vi "CC Quad Image Viewer.vi"(11 "Files":path[](array[path])) -> ()   [LabVIEW 2024]
uses:
  <vilib>/Utility/miscctls.llb/LVCursorListTypeDef.ctl
panel:
  in  "Transpose 1":bool
  out "Detector 1":sgl[][](graph)
  in  "Transpose 3":bool
  out "Detector 3":sgl[][](graph)
  in  "Transpose 2":bool
  out "Detector 2":sgl[][](graph)
  in  "Transpose 4":bool
  out "Detector 4":sgl[][](graph)
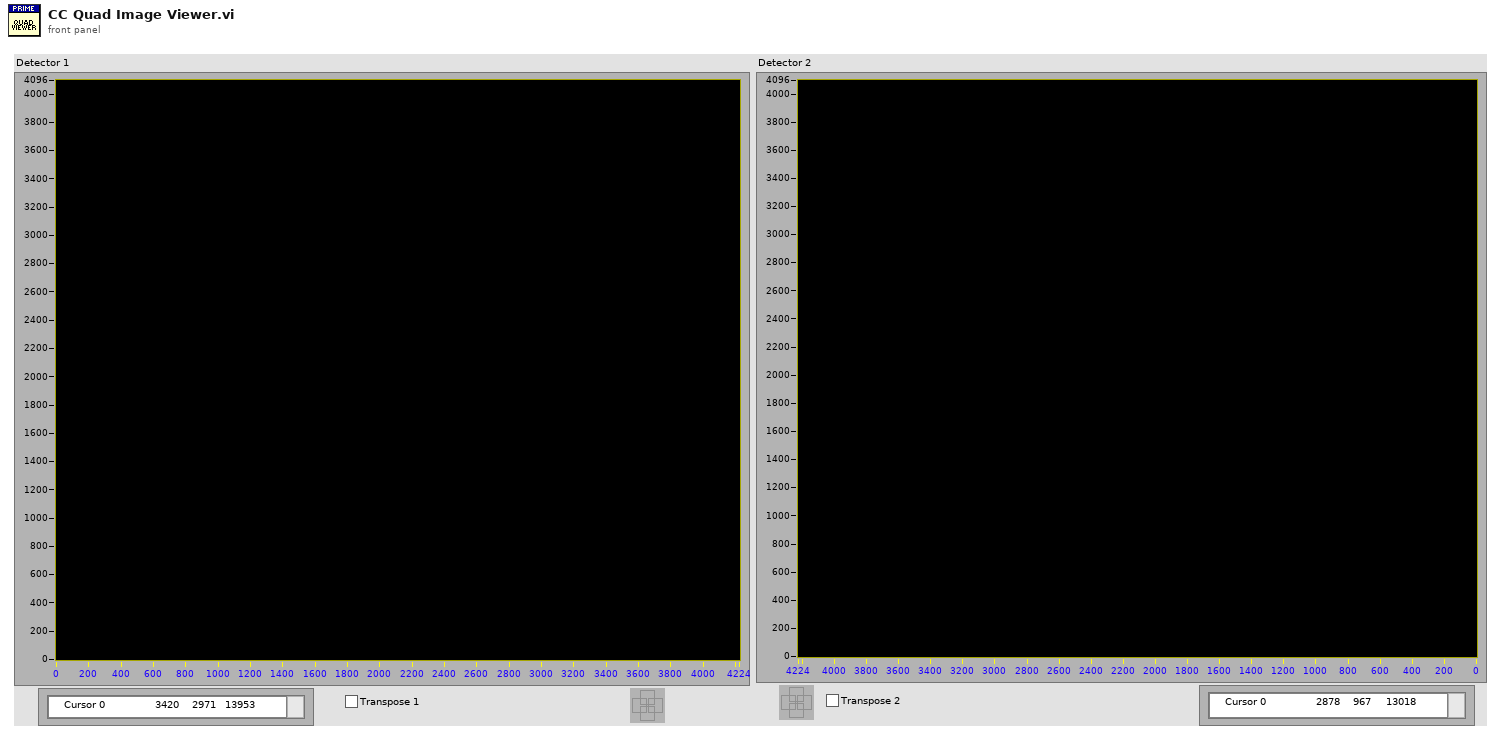
[diagram p1: front panel]
types:
  T1 = cluster{"state":refnum<user-event>, "plots":refnum<vi>[]}
  T2 = typedef "LVCursorListTypeDef.ctl" = cluster{"Name":string, "Color":u32, "Style":u8, "Point Style":u8, "Name Visible":bool, "Allow Drag":bool, "Cursor Mode":u32, "Plot":i32, "Index":i32, "Position":cluster{"X":dbl, "Y":dbl}, "X Scale":u32, "Y Scale":u32, "Watch Plots":i32[], "Watch All Plots":bool, "Plot Area":i32, "Label Offset":cluster{"X":dbl, "Y":dbl}}[]
  T3 = typedef "LVRectTypeDef.ctl" = cluster{"Left":i16, "Top":i16, "Right":i16, "Bottom":i16}
  T4 = typedef "CC cluster  Viewer Image Order.ctl" = cluster{"Top Left":i32, "Top Right":i32, "Bottom Left":i32, "Bottom Right":i32}
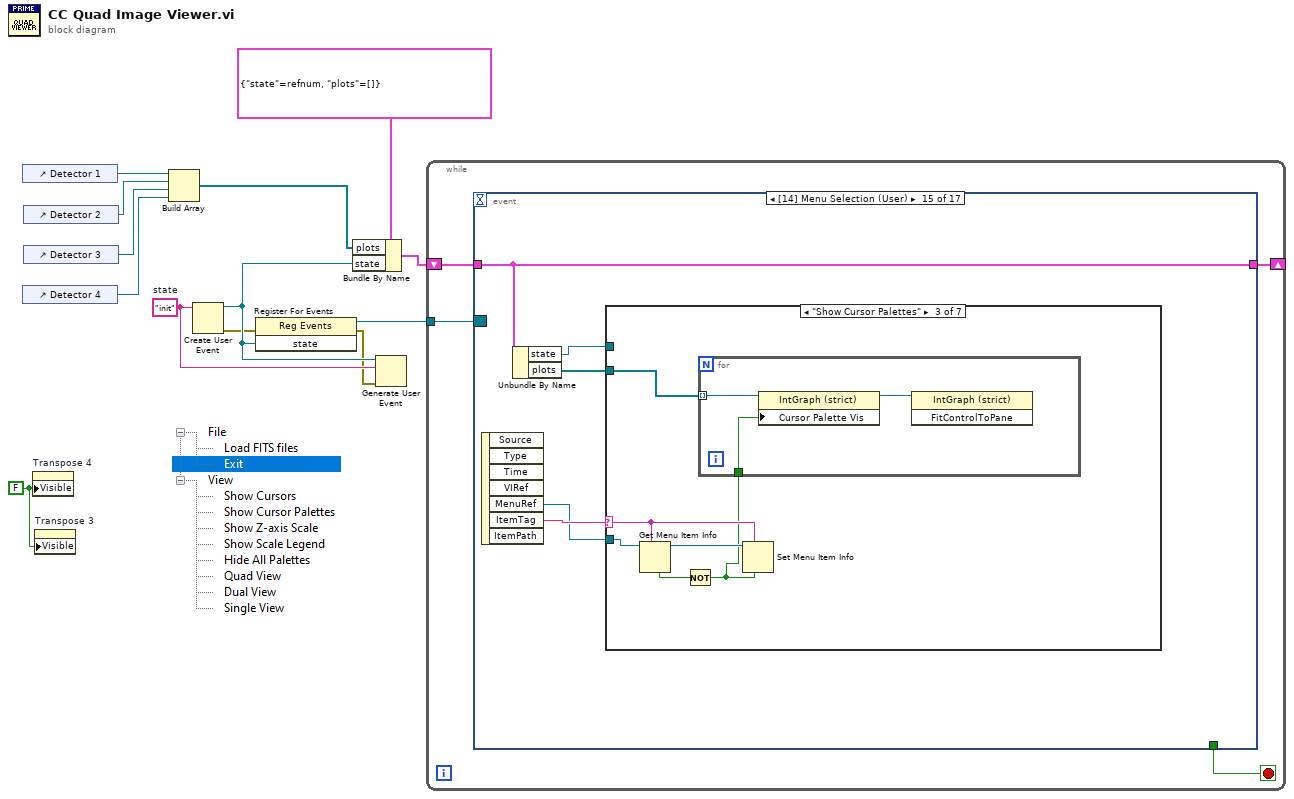
[diagram p0: block diagram]
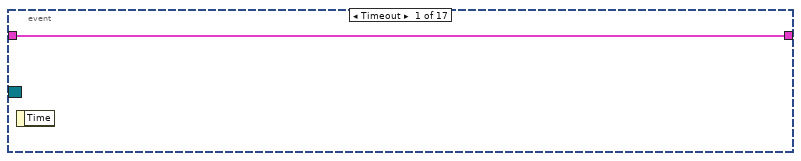
[diagram p2: hidden frame]
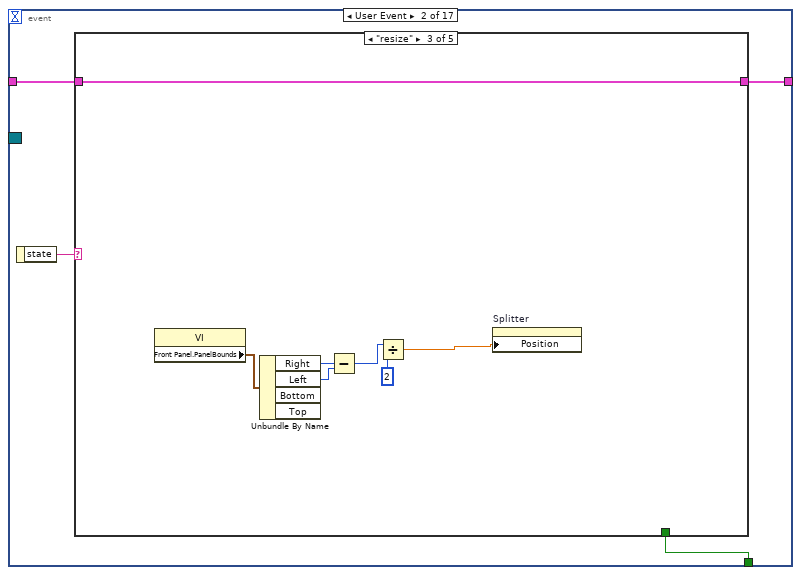
[diagram p3: hidden frame]
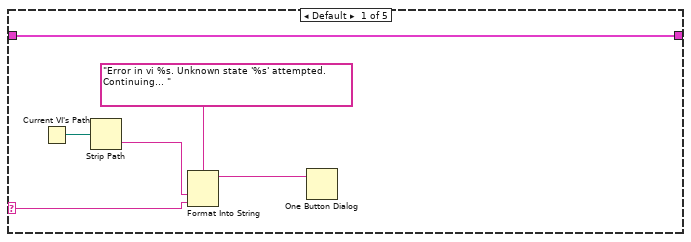
[diagram p4: hidden frame]
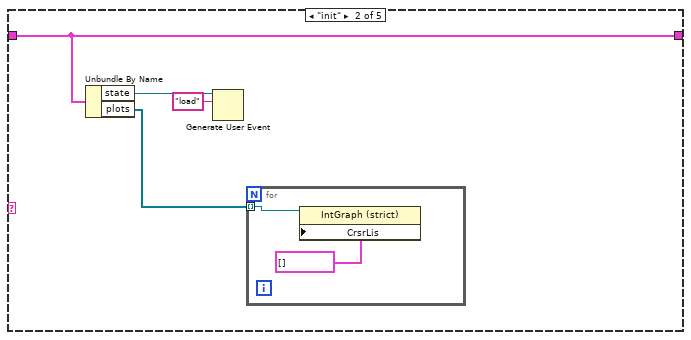
[diagram p5: hidden frame]
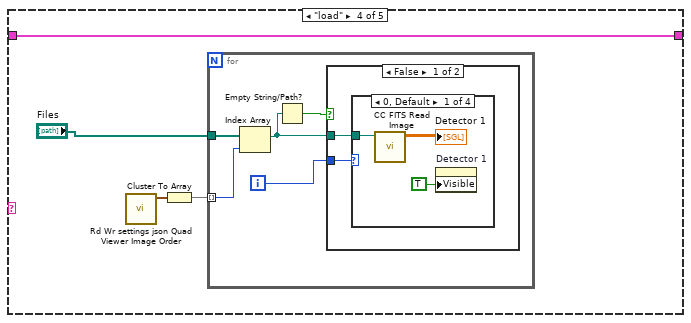
[diagram p6: hidden frame]
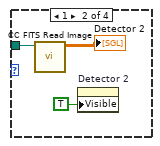
[diagram p7: hidden frame]
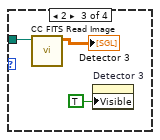
[diagram p8: hidden frame]
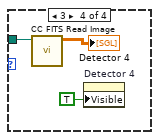
[diagram p9: hidden frame]
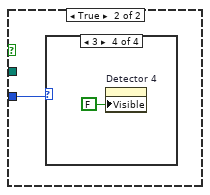
[diagram p10: hidden frame]
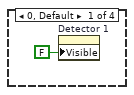
[diagram p11: hidden frame]
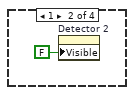
[diagram p12: hidden frame]
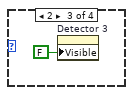
[diagram p13: hidden frame]
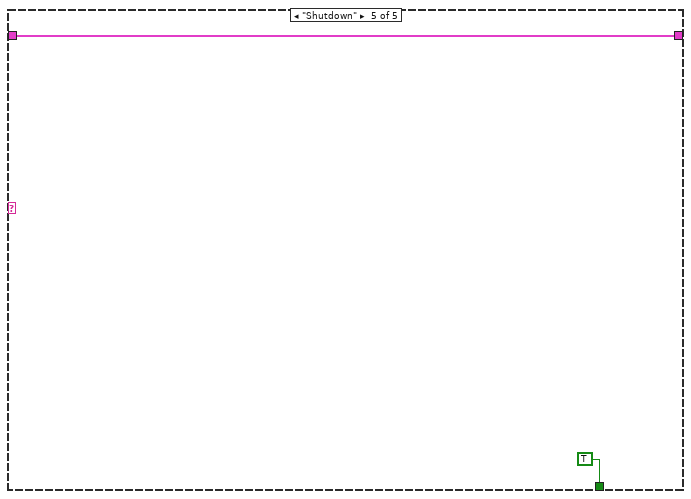
[diagram p14: hidden frame]
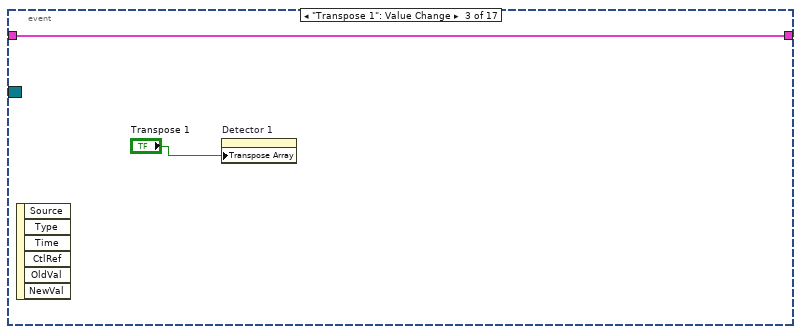
[diagram p15: hidden frame]
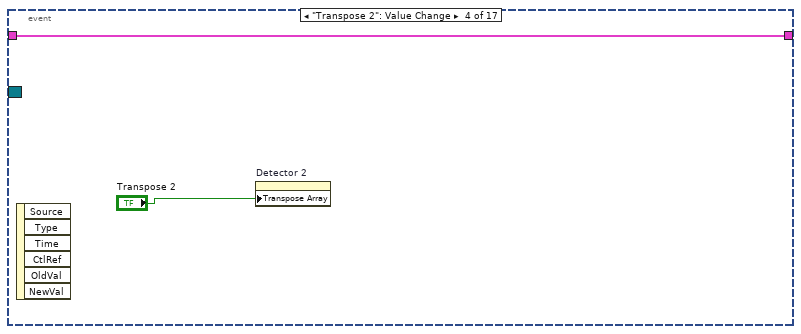
[diagram p16: hidden frame]
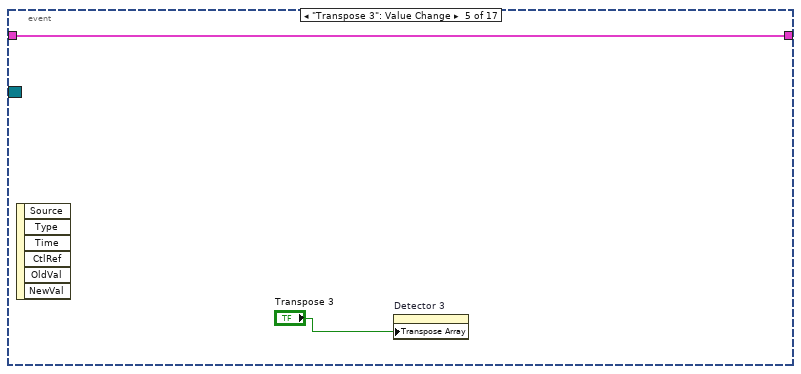
[diagram p17: hidden frame]
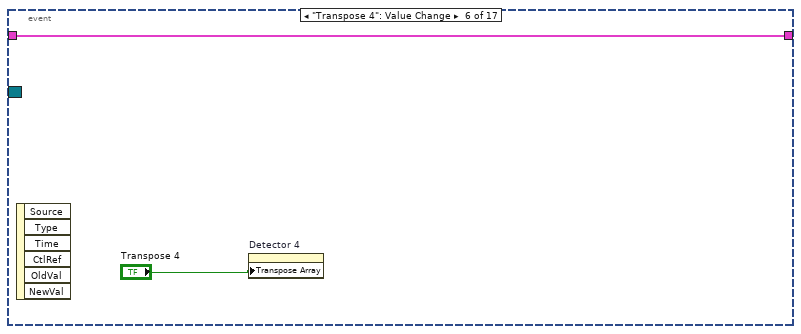
[diagram p18: hidden frame]
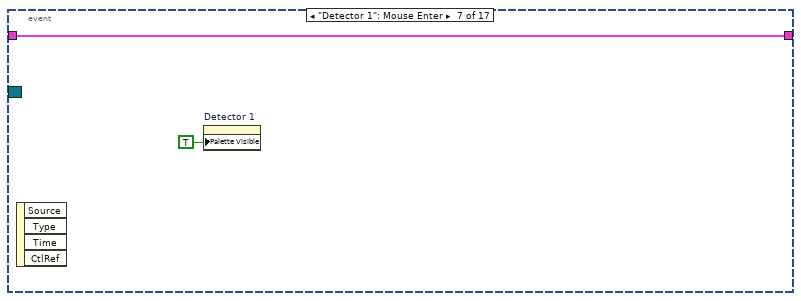
[diagram p19: hidden frame]
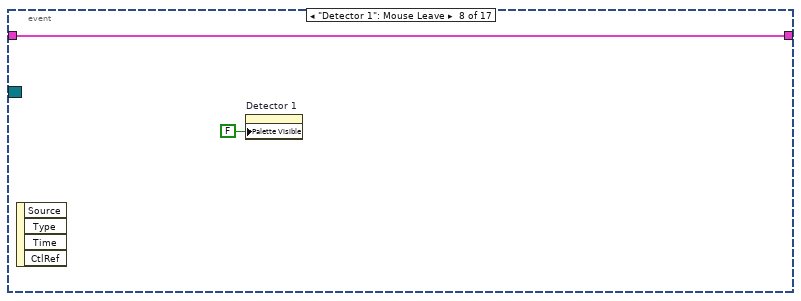
[diagram p20: hidden frame]
diagram:
  w1 = FALSE ("Visible")
  w9 = "init"  # state
  n1 = control-ref of="Detector 1"() -> (w6:refnum<vi>)
  n2 = control-ref of="Detector 4"() -> (w3:refnum<vi>)
  n3 = control-ref of="Detector 2"() -> (w5:refnum<vi>)
  n4 = control-ref of="Detector 3"() -> (w4:refnum<vi>)
  n5 = property on="Transpose 4" class="Bool (strict)"("Visible"=w1) -> ()  [unwired: 2 in, 2 out]
  n6 = property on="Transpose 3" class="Bool (strict)"("Visible"=w1) -> ()  [unwired: 2 in, 2 out]
  n7 = Build Array(w6, w5, w4, w3) -> (w2:refnum<vi>[])
  n8 = Create User Event(user event datatype=w9) -> (user event=w11:refnum<user-event>, error out=w7:errorcluster)  [unwired: 1 in]
  n9 = register-events(error in=w7, w11) -> (reference out=w10:refnum<event-registration>, error out=w8:errorcluster)  [unwired: 1 in]
  n10 = Bundle By Name(cluster=T1 {"state"=refnum, "plots"=[]}, "plots"=w2, "state"=w11) -> (w12:T1)
  n11 = Generate User Event(user event=w11, event data cluster=w9, error in=w8) -> ()  [unwired: 1 in, 2 out]
  n12 = while {
    tunnel: w10 -> [w17]
    shift-right: [w15] -> _
    shift-left: w12 -> [w16]
    stop <- w14 stop-if-true
    n13 = event shown="[14] Menu Selection (User)" {
      selector: w17 -> [_ _ _ _ _ _ _ _ _ _ _ _ _ _ _ _ _]
      dyn-events: _ -> [_ _ _ _ _ _ _ _ _ _ _ _ _ _ _ _ _]
      timeout: _ -> [_ _ _ _ _ _ _ _ _ _ _ _ _ _ _ _ _]
      tunnel: w16 -> [w18 w21 w73 w75 w77 w79 w81 w83 w85 w87 w89 w91 w93 w95 w99 w156 w160]
      tunnel: [w18 w20 w73 w75 w77 w79 w81 w83 w85 w87 w89 w91 w93 w95 w99 w156 w160] -> w15
      tunnel: [_ w19 _ _ _ _ _ _ _ _ _ _ _ _ _ _ _] -> w14
      event Timeout {
        n14 = event-data() -> ()  [unwired: 1 in, 1 out]
      }
      event User Event {
        n15 = event-data() -> ("state"=w22:string)  [unwired: 1 in]
        n16 = case shown="\"resize\"" w22 {
          selector: w22 -> [w27 _ _ _ _]
          tunnel: w21 -> [w23 w32 w41 w45 w71]
          tunnel: [w23 w32 w41 w45 w71] -> w20
          tunnel: [_ _ _ _ TRUE] -> w19
          frame Default {
            n17 = Current VI's Path() -> (path=w26:path)
            n18 = Strip Path(path=w26) -> (name=w25:string)  [unwired: 1 out]
            n19 = Format Into String(format string="Error in vi %s. Unknown state '%s' attempted. Continuing... ", w25, w27) -> (resulting string=w24:string)  [unwired: 2 in, 1 out]
            n20 = One Button Dialog(message=w24) -> ()  [unwired: 1 in, 1 out]
          }
          frame "init" {
            n21 = Unbundle By Name(w32) -> ("state"=w31:refnum<user-event>, "plots"=w29:refnum<vi>[])
            n22 = Generate User Event(user event=w31, event data cluster="load" ("event data")) -> ()  [unwired: 2 in, 2 out]
            n23 = for {
              tunnel: w29 -> [w34] mode=indexing
              n24 = property class="IntGraph (strict)"(reference=w34, "CrsrLis"=T2 [] ("Cursor List")) -> ()  [unwired: 1 in, 2 out]
            }
          }
          frame "resize" {
            n25 = property class="VI"() -> ("Front Panel.PanelBounds"=w39:T3)  [unwired: 2 in, 2 out]
            n26 = Unbundle By Name(w39) -> ("Right"=w38:i16, "Left"=w37:i16)  [unwired: 2 out]
            n27 = Subtract(x=w38, y=w37) -> (x-y=w36:i16)
            n28 = Divide(x=w36, y=2) -> (x/y=w35:dbl)
            n29 = property on="Splitter" class="Splitter"("Position"=w35) -> ()  [unwired: 2 in, 2 out]
          }
          frame "load" {
            n30 = call "Rd Wr settings json Quad Viewer Image Order.vi"() -> ("Image Order"=w43:T4)  [unwired: 10 in, 1 out]
            n31 = Cluster To Array(cluster=w43) -> (array=w42:i32[])
            n32 = for {
              tunnel: "Files" -> [w49]
              tunnel: w42 -> [w48] mode=indexing
              i -> [w50]
              n33 = Index Array(array=w49, index=w48) -> (element=w47:path)
              n34 = Empty String/Path?(string/path=w47) -> (empty?=w46:bool)
              n35 = case shown="False" w46 {
                tunnel: w50 -> [w52 w65]
                tunnel: w47 -> [w51 _]
                frame False {
                  n36 = case shown="0, Default" w52 {
                    tunnel: w51 -> [w55 w58 w61 w64]
                    frame 0, Default {
                      n37 = call "CC FITS Read Image.vi"("FITS File Path"=w55) -> ("Image"=→"Detector 1":sgl[][])  [unwired: 9 in, 1 out]
                      n38 = property on="Detector 1" class="IntGraph (strict)"("Visible"=TRUE) -> ()  [unwired: 2 in, 2 out]
                    }
                    frame 1 {
                      n39 = call "CC FITS Read Image.vi"("FITS File Path"=w58) -> ("Image"=→"Detector 2":sgl[][])  [unwired: 9 in, 1 out]
                      n40 = property on="Detector 2" class="IntGraph (strict)"("Visible"=TRUE) -> ()  [unwired: 2 in, 2 out]
                    }
                    frame 2 {
                      n41 = call "CC FITS Read Image.vi"("FITS File Path"=w61) -> ("Image"=→"Detector 3":sgl[][])  [unwired: 9 in, 1 out]
                      n42 = property on="Detector 3" class="IntGraph (strict)"("Visible"=TRUE) -> ()  [unwired: 2 in, 2 out]
                    }
                    frame 3 {
                      n43 = call "CC FITS Read Image.vi"("FITS File Path"=w64) -> ("Image"=→"Detector 4":sgl[][])  [unwired: 9 in, 1 out]
                      n44 = property on="Detector 4" class="IntGraph (strict)"("Visible"=TRUE) -> ()  [unwired: 2 in, 2 out]
                    }
                  }
                }
                frame True {
                  n45 = case shown="3" w65 {
                    frame 0, Default {
                      n46 = property on="Detector 1" class="IntGraph (strict)"("Visible"=FALSE) -> ()  [unwired: 2 in, 2 out]
                    }
                    frame 1 {
                      n47 = property on="Detector 2" class="IntGraph (strict)"("Visible"=FALSE) -> ()  [unwired: 2 in, 2 out]
                    }
                    frame 2 {
                      n48 = property on="Detector 3" class="IntGraph (strict)"("Visible"=FALSE) -> ()  [unwired: 2 in, 2 out]
                    }
                    frame 3 {
                      n49 = property on="Detector 4" class="IntGraph (strict)"("Visible"=FALSE) -> ()  [unwired: 2 in, 2 out]
                    }
                  }
                }
              }
            }
          }
          frame "Shutdown" {
          }
        }
      }
      event "Transpose 1": Value Change {
        n50 = event-data() -> ()  [unwired: 1 in, 6 out]
        n51 = property on="Detector 1" class="IntGraph (strict)"("Transpose Array"="Transpose 1") -> ()  [unwired: 2 in, 2 out]
      }
      event "Transpose 2": Value Change {
        n52 = event-data() -> ()  [unwired: 1 in, 6 out]
        n53 = property on="Detector 2" class="IntGraph (strict)"("Transpose Array"="Transpose 2") -> ()  [unwired: 2 in, 2 out]
      }
      event "Transpose 3": Value Change {
        n54 = event-data() -> ()  [unwired: 1 in, 6 out]
        n55 = property on="Detector 3" class="IntGraph (strict)"("Transpose Array"="Transpose 3") -> ()  [unwired: 2 in, 2 out]
      }
      event "Transpose 4": Value Change {
        n56 = event-data() -> ()  [unwired: 1 in, 6 out]
        n57 = property on="Detector 4" class="IntGraph (strict)"("Transpose Array"="Transpose 4") -> ()  [unwired: 2 in, 2 out]
      }
      event "Detector 1": Mouse Enter {
        n58 = event-data() -> ()  [unwired: 1 in, 4 out]
        n59 = property on="Detector 1" class="IntGraph (strict)"("Palette Visible"=TRUE ("Palette:Visible")) -> ()  [unwired: 2 in, 2 out]
      }
      event "Detector 1": Mouse Leave {
        n60 = event-data() -> ()  [unwired: 1 in, 4 out]
        n61 = property on="Detector 1" class="IntGraph (strict)"("Palette Visible"=FALSE ("Palette:Visible")) -> ()  [unwired: 2 in, 2 out]
      }
      event "Detector 2": Mouse Enter {
        n62 = event-data() -> ()  [unwired: 1 in, 4 out]
        n63 = property on="Detector 2" class="IntGraph (strict)"("Palette Visible"=TRUE ("Palette:Visible")) -> ()  [unwired: 2 in, 2 out]
      }
      event "Detector 2": Mouse Leave {
        n64 = event-data() -> ()  [unwired: 1 in, 4 out]
        n65 = property on="Detector 2" class="IntGraph (strict)"("Palette Visible"=FALSE ("Palette:Visible")) -> ()  [unwired: 2 in, 2 out]
      }
      event "Detector 3": Mouse Enter {
        n66 = event-data() -> ()  [unwired: 1 in, 4 out]
        n67 = property on="Detector 3" class="IntGraph (strict)"("Palette Visible"=TRUE ("Palette:Visible")) -> ()  [unwired: 2 in, 2 out]
      }
      event "Detector 3": Mouse Leave {
        n68 = event-data() -> ()  [unwired: 1 in, 4 out]
        n69 = property on="Detector 3" class="IntGraph (strict)"("Palette Visible"=FALSE ("Palette:Visible")) -> ()  [unwired: 2 in, 2 out]
      }
      event "Detector 4": Mouse Enter {
        n70 = event-data() -> ()  [unwired: 1 in, 4 out]
        n71 = property on="Detector 4" class="IntGraph (strict)"("Palette Visible"=TRUE ("Palette:Visible")) -> ()  [unwired: 2 in, 2 out]
      }
      event "Detector 4": Mouse Leave {
        n72 = event-data() -> ()  [unwired: 1 in, 4 out]
        n73 = property on="Detector 4" class="IntGraph (strict)"("Palette Visible"=FALSE ("Palette:Visible")) -> ()  [unwired: 2 in, 2 out]
      }
      event Menu Selection (User) {
        n74 = event-data() -> ("MenuRef"=w97:refnum<k9>, "ItemTag"=w100:string)  [unwired: 1 in, 5 out]
        n75 = Unbundle By Name(w99) -> ("state"=w96:refnum<user-event>, "plots"=w98:refnum<vi>[])
        n76 = case shown="\"Show Cursor Palettes\"" w100 {
          selector: w100 -> [_ w103 w119 w128 w137 w146 _]
          tunnel: w98 -> [_ w106 w116 w125 w134 w143 _]
          tunnel: w97 -> [_ w102 w120 w129 w138 w149 _]
          tunnel: w96 -> [_ _ _ _ _ _ w154]
          frame "False", Default {
          }
          frame "Show Cursors" {
            n77 = Get Menu Item Info(7:w103, 11:w102) -> (3:w105:refnum<k9>, 4:w104:bool)  [unwired: 1 in, 5 out]
            n78 = Not(x=w104) -> (.not. x?=w101:bool)
            n79 = for {
              tunnel: w106 -> [w111] mode=indexing
              tunnel: w101 -> [w107]
              n80 = property class="IntGraph (strict)"(reference=w111) -> (reference out=w108:refnum<vi>, "CrsrLis"=w110:T2)  [unwired: 1 in, 1 out]
              n81 = Array Size(array=w110) -> (size(s)=w109:i32)
              n82 = for {
                N: w109 -> [_]
                tunnel: w108 -> [w114]
                tunnel: w107 -> [w112]
                i -> [w113]
                n83 = property class="IntGraph (strict)"(reference=w114, "Active Cursor"=w113, "Cursor.Visible"=w112) -> ()  [unwired: 1 in, 2 out]
              }
            }
            n84 = Set Menu Item Info(6:w101, 7:w103, 11:w105) -> ()  [unwired: 4 in, 2 out]
          }
          frame "Show Cursor Palettes" {
            n85 = Get Menu Item Info(7:w119, 11:w120) -> (3:w118:refnum<k9>, 4:w117:bool)  [unwired: 1 in, 5 out]
            n86 = Not(x=w117) -> (.not. x?=w115:bool)
            n87 = for {
              tunnel: w116 -> [w123] mode=indexing
              tunnel: w115 -> [w122]
              n88 = property class="IntGraph (strict)"(reference=w123, "Cursor Palette Vis"=w122) -> (reference out=w121:refnum<vi>)  [unwired: 1 in, 1 out]
              n89 = invoke class="IntGraph (strict)" method="FitControlToPane"(reference=w121) -> ()  [unwired: 2 in, 3 out]
            }
            n90 = Set Menu Item Info(6:w115, 7:w119, 11:w118) -> ()  [unwired: 4 in, 2 out]
          }
          frame "Show Z-axis Scale" {
            n91 = Get Menu Item Info(7:w128, 11:w129) -> (3:w127:refnum<k9>, 4:w126:bool)  [unwired: 1 in, 5 out]
            n92 = Not(x=w126) -> (.not. x?=w124:bool)
            n93 = for {
              tunnel: w125 -> [w132] mode=indexing
              tunnel: w124 -> [w131]
              n94 = property class="IntGraph (strict)"(reference=w132, "ZScale.Visible"=w131, "ZScale.RampVis"=w131) -> (reference out=w130:refnum<vi>)  [unwired: 1 in, 1 out]
              n95 = invoke class="IntGraph (strict)" method="FitControlToPane"(reference=w130) -> ()  [unwired: 2 in, 3 out]
            }
            n96 = Set Menu Item Info(6:w124, 7:w128, 11:w127) -> ()  [unwired: 4 in, 2 out]
          }
          frame "Show Scale Legend" {
            n97 = Get Menu Item Info(7:w137, 11:w138) -> (3:w136:refnum<k9>, 4:w135:bool)  [unwired: 1 in, 5 out]
            n98 = Not(x=w135) -> (.not. x?=w133:bool)
            n99 = for {
              tunnel: w134 -> [w141] mode=indexing
              tunnel: w133 -> [w140]
              n100 = property class="IntGraph (strict)"(reference=w141, "ScaleLegendVis"=w140) -> (reference out=w139:refnum<vi>)  [unwired: 1 in, 1 out]
              n101 = invoke class="IntGraph (strict)" method="FitControlToPane"(reference=w139) -> ()  [unwired: 2 in, 3 out]
            }
            n102 = Set Menu Item Info(6:w133, 7:w137, 11:w136) -> ()  [unwired: 4 in, 2 out]
          }
          frame "Hide All Palettes" {
            n103 = Get Menu Item Info(7:w146, 11:w149) -> (2:w147:string, 3:w148:refnum<k9>)  [unwired: 1 in, 5 out]
            n104 = Not Equal?(x=w146, y=w147) -> (x != y?=w142:bool)
            n105 = for {
              tunnel: w143 -> [w152] mode=indexing
              tunnel: w142 -> [w150]
              n106 = property class="IntGraph (strict)"(reference=w152, "ScaleLegendVis"=w150, "ZScale.Visible"=w150, "ZScale.RampVis"=w150, "ScaleLegendVis"=w150, "Cursor Palette Vis"=w150, "Palette Visible"=w150) -> (reference out=w151:refnum<vi>)  [unwired: 1 in, 1 out]
              n107 = invoke class="IntGraph (strict)" method="FitControlToPane"(reference=w151) -> ()  [unwired: 2 in, 3 out]
            }
            n108 = Select(t=w146, s=w142, f="Show Palettes") -> (s? t:f=w145:string)
            n109 = Set Menu Item Info(7:w146, 10:w145, 11:w148) -> ()  [unwired: 4 in, 2 out]
          }
          frame "Exit" {
            n110 = Generate User Event(user event=w154, event data cluster="Shutdown" ("event data")) -> ()  [unwired: 2 in, 2 out]
          }
        }
      }
      event Panel Close {
        n111 = event-data() -> ()  [unwired: 1 in, 4 out]
        n112 = Unbundle By Name(w156) -> ("state"=w155:refnum<user-event>)
        n113 = Generate User Event(user event=w155, event data cluster="Shutdown" ("event data")) -> ()  [unwired: 2 in, 2 out]
      }
      event Panel Resize {
        n114 = event-data() -> ()  [unwired: 1 in, 8 out]
        n115 = Unbundle By Name(w160) -> ("state"=w159:refnum<user-event>)
        n116 = Generate User Event(user event=w159, event data cluster="resize" ("event data")) -> ()  [unwired: 2 in, 2 out]
      }
    }
  }
